vi "Receive TX Message.vi"(8 "error in (no error)":errorcluster, 10 "timeout in ms":i32=5, 11 "RxTx in":refnum<class "RxTx.lvclass">) -> (0 "error out":errorcluster, 3 "RxTx out":refnum<class "RxTx.lvclass">)   [LabVIEW 2018, in "RxTx.lvclass"]
uses:
  RxTx.lvclass
  RxTx.lvclass/RxTx.ctl
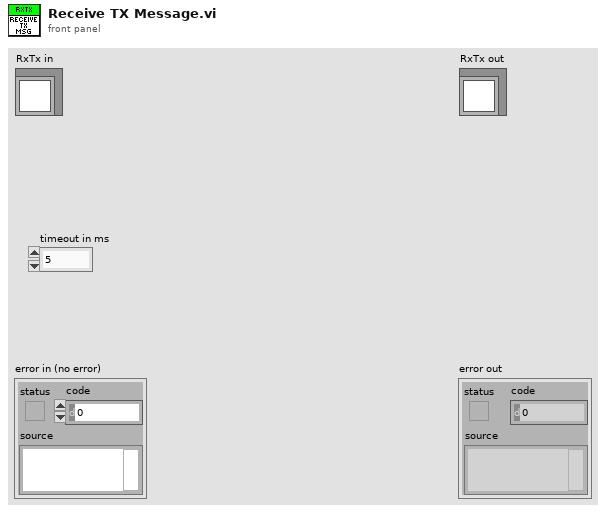
[diagram p1: front panel]
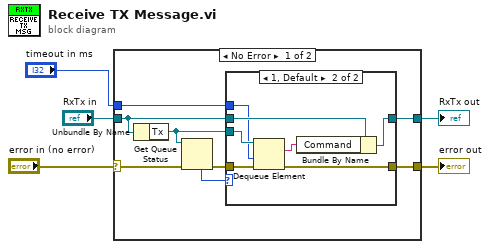
[diagram p0: block diagram]
diagram:
  n1 = case shown="No Error" "error in (no error)" {
    selector: "error in (no error)" -> [w8 w24]
    tunnel: [w6 w24] -> w3
    tunnel: [w12 w23] -> w2
    tunnel: "RxTx in" -> [w13 w23]
    tunnel: "timeout in ms" -> [w11 _]
    frame No Error {
      n2 = Unbundle By Name(w13) -> ("Tx"=w9:refnum<queue>)
      n3 = Get Queue Status(queue=w9, error in (no error)=w8) -> (error out=w7:errorcluster, # elements in queue=w10:i32)  [unwired: 1 in, 6 out]
      n4 = case shown="1, Default" w10 {
        tunnel: w9 -> [_ w22]
        tunnel: w13 -> [w14 w21]
        tunnel: [w14 w20] -> w12
        tunnel: w11 -> [_ w18]
        tunnel: w7 -> [w15 w17]
        tunnel: [w15 w16] -> w6
        frame 0 {
        }
        frame 1, Default {
          n5 = Dequeue Element(queue=w22, timeout in ms (-1)=w18, error in (no error)=w17) -> (element=w19:string, error out=w16:errorcluster)  [unwired: 2 out]
          n6 = Bundle By Name(cluster=w21, "Command"=w19) -> (w20:refnum<class "RxTx.lvclass">)
        }
      }
    }
    frame Error {
    }
  }
  "error out" <- w3
  "RxTx out" <- w2
